vi "SeCrTs-AI_Read_P3.vi"(5 "Data FIFO Ref":T1, 6 "error in (no error)":errorcluster, 7 "Numeric":dbl=10.0, 9 "AI_Task":refnum<k21>) -> (0 "error out":errorcluster, 3 "task out":refnum<k21>)   [LabVIEW 2022 SP3]
uses:
  RT Controls/SeCrTs-Data FIFO.ctl
  <vilib>/Platform/TimedLoop/XDataNode/timing_clust.ctl
  <vilib>/Platform/TimedLoop/XDataNode/nitl_modes.ctl
  <vilib>/Platform/TimedLoop/XDataNode/wakeup.ctl
  <vilib>/DAQmx/read.llb/DAQmx Read (Analog 1D Wfm NChan NSamp).vi
  <vilib>/DAQmx/miscellaneous.llb/DAQmx Fill In Error Info.vi
  <vilib>/platform/TimedLoop/XDataNode/XDataNode.xnode
  <vilib>/Platform/TimedLoop/XDataNode/XDNodeRunTimeDep.lvlib
panel:
  out "overflow?":bool
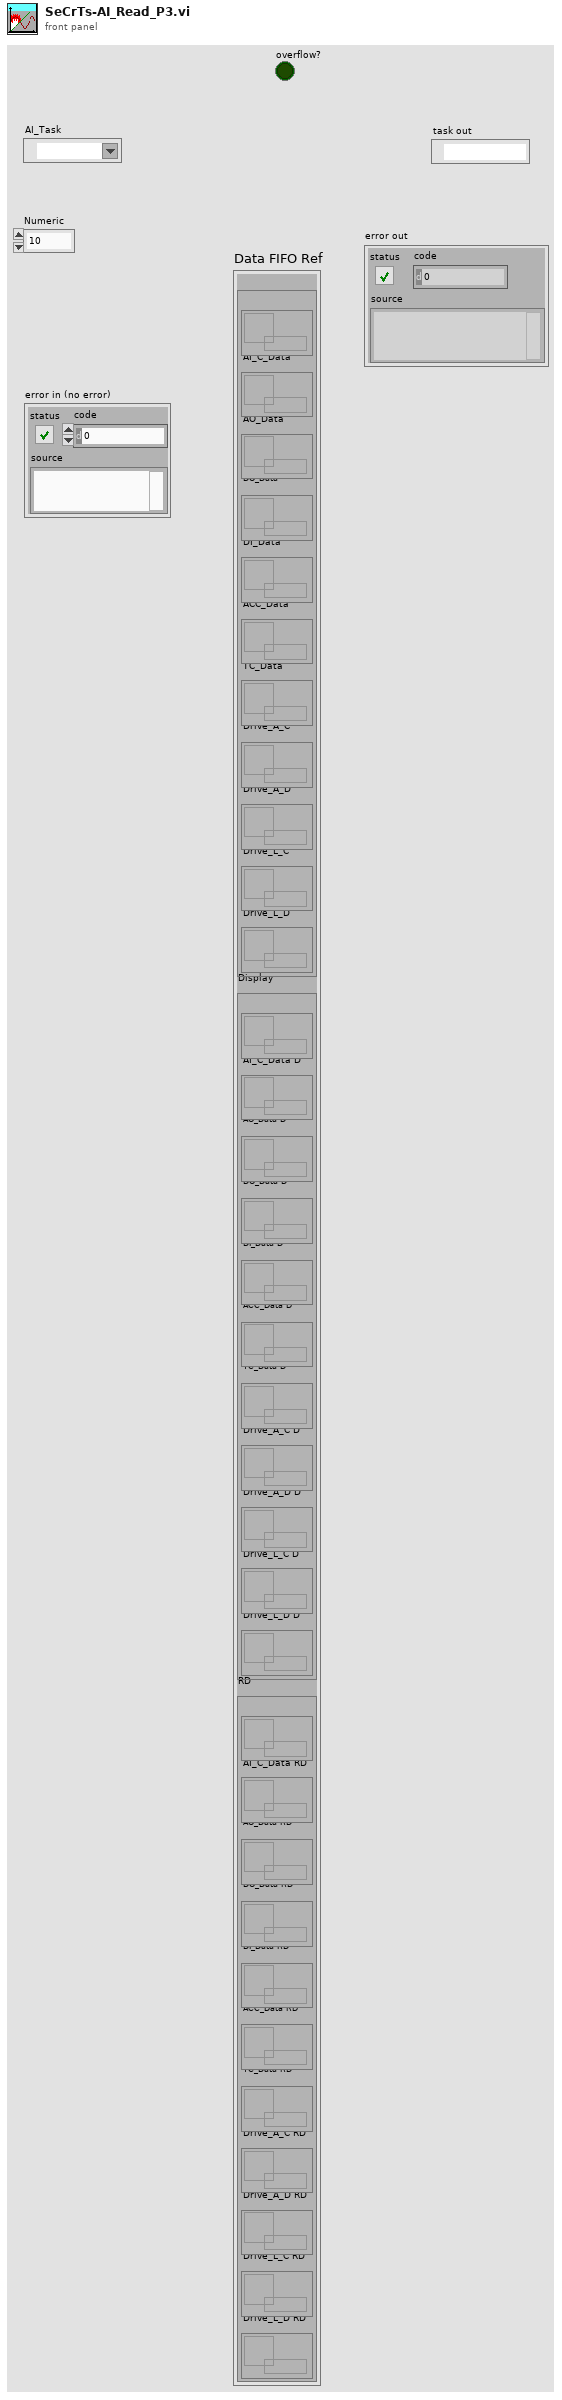
[diagram p1: front panel]
types:
  T1 = typedef "SeCrTs-Data FIFO.ctl" = cluster{"Control":cluster{"AI_V_Data":refnum<queue>, "AI_C_Data":refnum<queue>, "AO_Data":refnum<queue>, "DO_Data":refnum<queue>, "DI_Data":refnum<queue>, "ACC_Data":refnum<queue>, "TC_Data":refnum<queue>, "Drive_A_C":refnum<queue>, "Drive_A_D":refnum<queue>, "Drive_L_C":refnum<queue>, "Drive_L_D":refnum<queue>}, "Display":cluster{"AI_V_Data D":refnum<queue>, "AI_C_Data D":refnum<queue>, "AO_Data D":refnum<queue>, "DO_Data D":refnum<queue>, "DI_Data D":refnum<queue>, "ACC_Data D":refnum<queue>, "TC_Data D":refnum<queue>, "Drive_A_C D":refnum<queue>, "Drive_A_D D":refnum<queue>, "Drive_L_C D":refnum<queue>, "Drive_L_D D":refnum<queue>}, "RD":cluster{"AI_V_Data RD":refnum<queue>, "AI_C_Data RD":refnum<queue>, "AO_Data RD":refnum<queue>, "DO_Data RD":refnum<queue>, "DI_Data RD":refnum<queue>, "ACC_Data RD":refnum<queue>, "TC_Data RD":refnum<queue>, "Drive_A_C RD":refnum<queue>, "Drive_A_D RD":refnum<queue>, "Drive_L_C RD":refnum<queue>, "Drive_L_D RD":refnum<queue>}}
  T2 = typedef "XDNodeRunTimeDep.lvlib/timing_clust.ctl" = cluster{"Expected End [f-1]":u64, "Actual End [f-1]":u64, "Finished Late? [f-1]":bool, "Expected End [i-1]":u64, "Actual End [i-1]":u64, "Finished Late? [i-1]":bool, "Expected Start [i]":u64, "Actual Start [i]":u64, "Expected Start [f]":u64, "Actual Start [f]":u64, "Source Name":string, "Structure Name":string, "Period":i64, "Deadline":i64, "Offset":i64, "Start":i64, "Priority":i32, "Timeout":i32, "Mode":T3, "Wakeup Reason":T4, "Error":errorcluster, "Source Type":string, "Secondary Source Type":string, "Global End Time":u64, "Global Start Time":u64, "Frame Duration":u64, "Iteration Duration":u64, "Assigned CPU":i32, "I/O Scan Engine Mode":u32}
  T3 = typedef "XDNodeRunTimeDep.lvlib/nitl_modes.ctl" = enum32{"No Change", "Process missed periods, maintain original phase", "Discard missed periods, maintain original phase", "Process missed periods, ignore original phase", "Discard missed periods, ignore original phase"}
  T4 = typedef "XDNodeRunTimeDep.lvlib/wakeup.ctl" = enum32{"Normal", "Aborted", "Asynchronous wakeup", "Timing source error", "Timed loop error", "Timeout"}
  T5 = enum16{"AI C", "AI V", "AO", "DI", "DO", "TC", "ACC", "DR L", "DR A"}
  T6 = enum16{"Init", "Read 'All'", "Read 'n'", "Read '1'", "Write '1'", "Write 'n'", "Write 'All'"}
  T7 = cluster{"Start DAQ":bool, "Stop DAQ":bool, "RT Stop":bool, "RT Exit":bool, "Start Seq":bool}
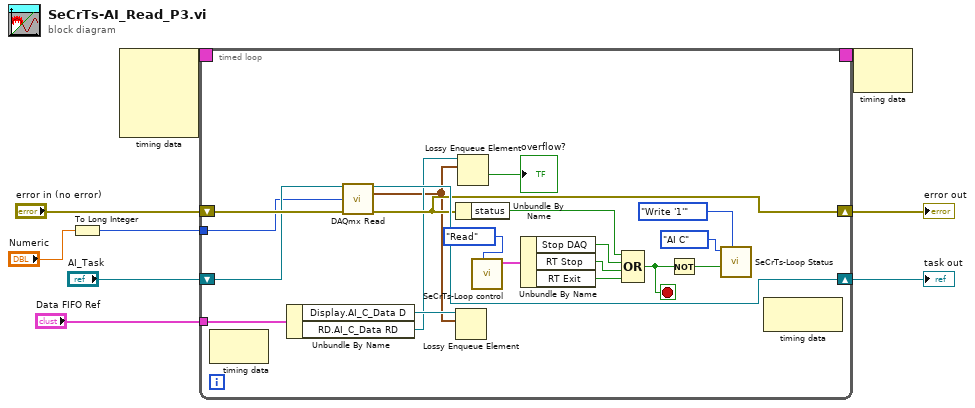
[diagram p0: block diagram]
diagram:
  n1 = To Long Integer(number="Numeric") -> (32bit integer=w5:i32)
  n2 = node-c288() -> (w2:T2)  [unwired: 4 in]
  n3 = timed-loop {
    tunnel: w5 -> [w17]
    tunnel: "Data FIFO Ref" -> [w14]
    shift-right: [w16] -> w4
    shift-left: "AI_Task" -> [w28]
    shift-right: [w15] -> w3
    shift-left: "error in (no error)" -> [w29]
    timing: w2 -> [_]
    timing-out: [_] -> w1
    stop <- w27 stop-if-true
    n4 = node-c288() -> ()  [unwired: 1 in, 1 out]
    n5 = Unbundle By Name(w14) -> ("Display.AI_C_Data D"=w13:refnum<queue>, "RD.AI_C_Data RD"=w12:refnum<queue>)
    n6 = call-poly <vilib>:"DAQmx Read.vi"("task/channels in"=w28, "number of samples per channel"=w17, "error in"=w29) -> ("task out"=w16:refnum<k21>, "data"=w11:waveform(dbl)[], "error out"=w15:errorcluster)  [unwired: 10 in]
    n7 = Unbundle By Name(w15) -> ("status"=w26:bool)
    n8 = Lossy Enqueue Element(queue=w13, element=w11) -> ()  [unwired: 1 in, 4 out]
    n9 = Lossy Enqueue Element(queue=w12, element=w11) -> (overflow?=→"overflow?":bool)  [unwired: 1 in, 3 out]
    n10 = call "SeCrTs-Loop control.vi"("Action"=enum16{"Init", "Write", "Read"}."Read") -> ("Loop Control out"=w25:T7)  [unwired: 9 in, 1 out]
    n11 = Unbundle By Name(w25) -> ("Stop DAQ"=w24:bool, "RT Stop"=w23:bool, "RT Exit"=w22:bool)
    n12 = Compound Arithmetic op=OR(w26, w24, w23, w22) -> (w27:bool)
    n13 = Not(x=w27) -> (.not. x?=w18:bool)
    n14 = call "SeCrTs-Loop Status.vi"("Option"=T6."Write '1'", "Status"=w18, "Loop"=T5."AI C") -> ()  [unwired: 6 in, 3 out]
    n15 = node-c288() -> ()  [unwired: 1 in, 1 out]
  }
  "task out" <- w4
  "error out" <- w3
  n16 = node-c288(w1) -> ()  [unwired: 1 out]
